vi "Solve2.vi"(8 "Error In":errorcluster, 11 "object in":refnum<class "2021_21.lvclass">) -> (0 "Error Out":errorcluster, 2 "Result":u64, 3 "object out":refnum<class "2021_21.lvclass">)   [LabVIEW 2020, in "2021_21.lvclass"]
uses:
  2021_21.lvclass
  2021_21.lvclass/2021_21.ctl
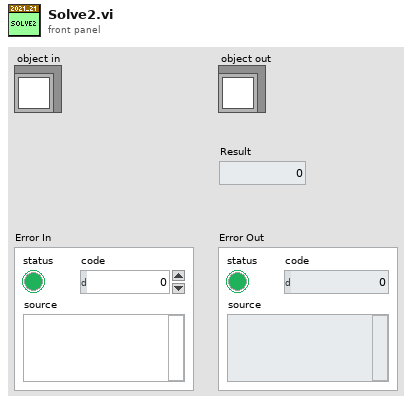
[diagram p1: front panel]
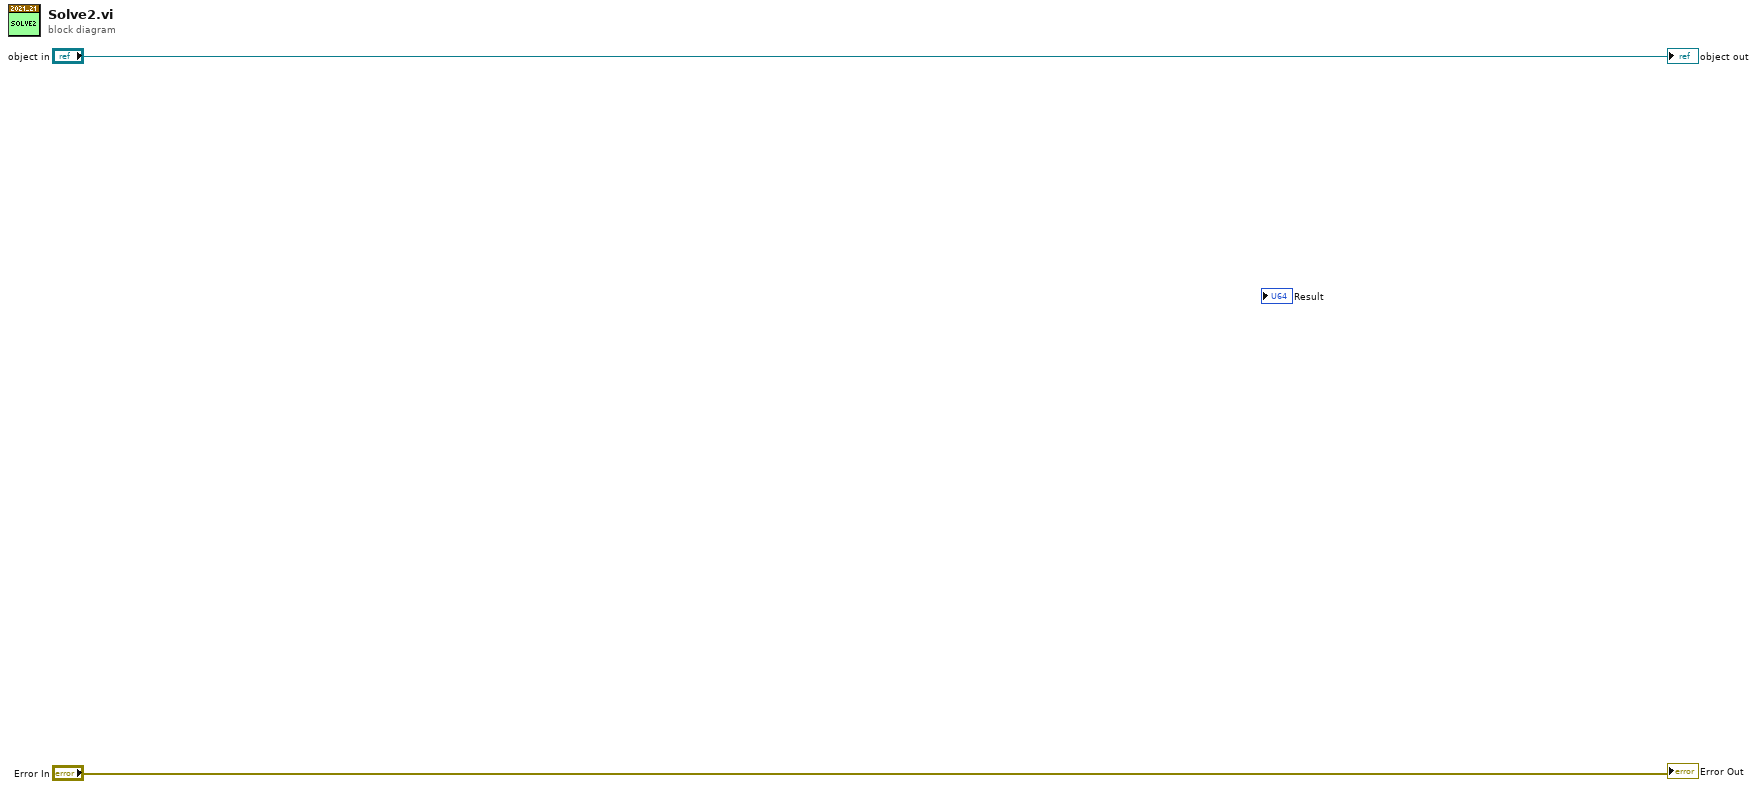
[diagram p0: block diagram]
diagram:
  "Error Out" <- "Error In"
  "object out" <- "object in"
